vi "Channel Settings to Digital.vi"(11 "channel settings":T1[](array[typedef])) -> (2 "channel default values":dbl[](array[numeric]), 3 "channel names":string[](array[string]))   [LabVIEW 2017, in "Scan Engine Scripting.lvlib"]
uses:
  Scan Engine Scripting.lvlib
  Modules/Mode Classes/Controls/digital channel settings.ctl
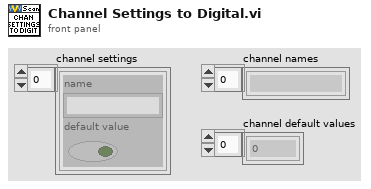
[diagram p1: front panel]
types:
  T1 = typedef "Scan Engine Scripting.lvlib/digital channel settings.ctl" = cluster{"name":string, "default value":bool}
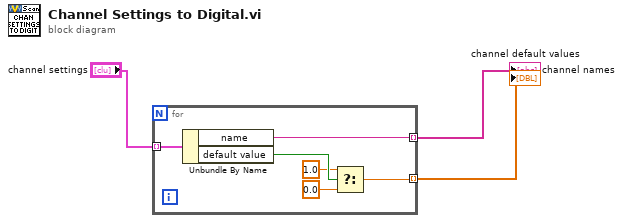
[diagram p0: block diagram]
diagram:
  n1 = for {
    tunnel: "channel settings" -> [w9] mode=indexing
    tunnel: [w8] -> w2 mode=indexing
    tunnel: [w4] -> w3 mode=indexing
    n2 = Unbundle By Name(w9) -> ("name"=w8:string, "default value"=w7:bool)
    n3 = Select(t=1.0, s=w7, f=0.0) -> (s? t:f=w4:dbl)
  }
  "channel default values" <- w3
  "channel names" <- w2
